vi "IsDwellComplete.vi"(11 "AutoData":T1) -> (1 "TimeRemaining":dbl, 2 "ElapsedTime":dbl, 3 "IsElapsed":bool)   [LabVIEW 2019, in "AutoMode.lvlib"]
uses:
  AutoMode.lvlib
  Cluster - AutoModeData.ctl
  MainController/Cluster - TestSettings.ctl
  MainController/Cluster - HardwareConfiguration.ctl
  MainController/Cluster - TestResults.ctl
  MainController/MainController.lvlib
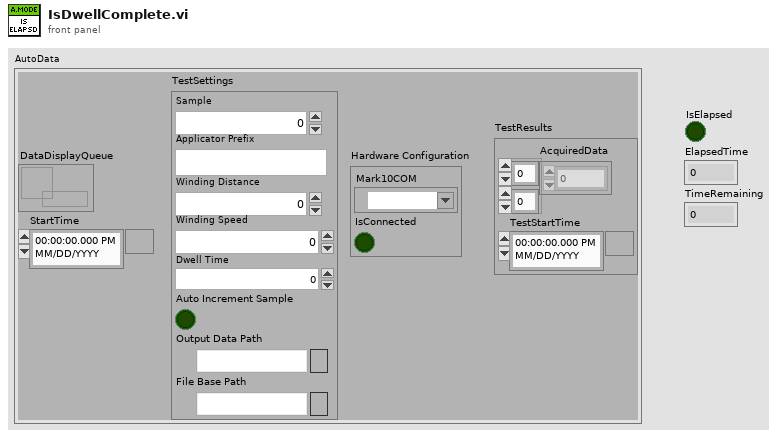
[diagram p1: front panel]
types:
  T1 = typedef "AutoMode.lvlib/Cluster - AutoModeData.ctl" = cluster{"DataDisplayQueue":refnum<queue>, "StartTime":timestamp, "TestSettings":T2, "Hardware Configuration":T3, "TestResults":T4}
  T2 = typedef "MainController.lvlib/Cluster - TestSettings.ctl" = cluster{"Sample":u32, "Applicator Prefix":string, "Winding Distance":dbl, "Winding Speed":dbl, "Dwell Time":dbl, "Auto Increment Sample":bool, "Output Data Path":path, "File Base Path":path}
  T3 = typedef "MainController.lvlib/Cluster - HardwareConfiguration.ctl" = cluster{"Mark10COM":refnum<visa-resource-name>, "IsConnected":bool}
  T4 = typedef "MainController.lvlib/Cluster - TestResults.ctl" = cluster{"AcquiredData":dbl[][], "TestStartTime":timestamp}
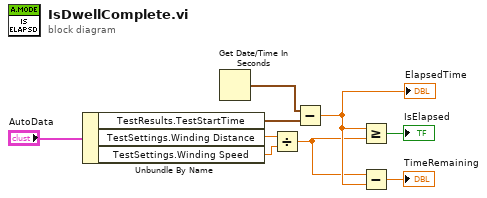
[diagram p0: block diagram]
diagram:
  n1 = Unbundle By Name("AutoData") -> ("TestResults.TestStartTime"=w8:timestamp, "TestSettings.Winding Distance"=w3:dbl, "TestSettings.Winding Speed"=w2:dbl)
  n2 = Get Date/Time In Seconds() -> (seconds since 1Jan1904=w7:timestamp)
  n3 = Divide(x=w3, y=w2) -> (x/y=w1:dbl)
  n4 = Subtract(x=w7, y=w8) -> (x-y=w5:dbl)
  "ElapsedTime" <- w5
  n5 = Greater Or Equal?(x=w5, y=w1) -> (x >= y?=→"IsElapsed":bool)
  n6 = Subtract(x=w1, y=w5) -> (x-y=→"TimeRemaining":dbl)
